vi "Motor Overheat detection.vi"() -> (0 "Array":string[](array[string]), 1 "Cascade Sensor":bool, 2 "Rhino Sensors":bool, 3 "Drivebase Sensors":bool)   [LabVIEW 2018]
uses:
  <vilib>/ptbypt/NI_PtbyPt.lvlib
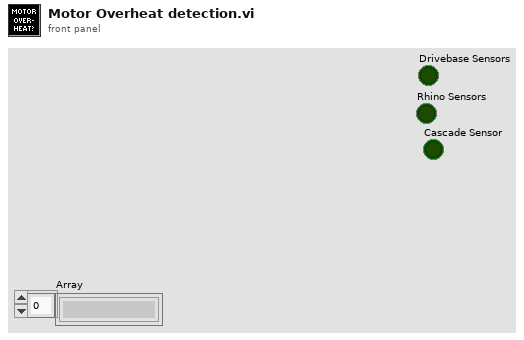
[diagram p1: front panel]
types:
  T1 = typedef "WPI_MotorControlDeviceRef.ctl" = cluster{"DeviceStatus":errorcluster, "Type":T2, "PWM":cluster{"PWM Channel":T3, "DeadBand":T4}, "CAN":cluster{"Device Number":u8, "SetOutput VI Ref":variant, "GetOutput VI Ref":variant, "Enable VI Ref":variant, "Disable VI Ref":variant, "Data":variant}, "Invert":bool, "DIO PWM":cluster{"PWM \"Enable\" Channel":T3, "DIOChannel":T5, "PWM Rate":dbl}}
  T2 = typedef "WPI_MotorControlType.ctl" = enum16{"PWM", "CAN", "DIO PWM"}
  T3 = typedef "FPGA_DIOPWMChannel.ctl" = enum8{"PWM 0", "PWM 1", "PWM 2", "PWM 3", "PWM 4", "PWM 5", "PWM 6", "PWM 7", "PWM 8", "PWM 9", "PWM MXP 0", "PWM MXP 1", "PWM MXP 2", "PWM MXP 3", "PWM MXP 4", "PWM MXP 5", "PWM MXP 6", "PWM MXP 7", "PWM MXP 8", "PWM MXP 9", "Invalid"}
  T4 = typedef "WPI_PWMDeadband.ctl" = cluster{"Name":string, "maxPositivePwm":i32, "minPositivePwm":i32, "centerPwm":i32, "maxNegativePwm":i32, "minNegativePwm":i32, "angularRange":u16}
  T5 = typedef "FPGA_DIOChannel.ctl" = enum8{"DIO 0", "DIO 1", "DIO 2", "DIO 3", "DIO 4", "DIO 5", "DIO 6", "DIO 7", "DIO 8", "DIO 9", "DIO MXP 0", "DIO MXP 1", "DIO MXP 2", "DIO MXP 3", "DIO MXP 4", "DIO MXP 5", "DIO MXP 6", "DIO MXP 7", "DIO MXP 8", "DIO MXP 9", "DIO MXP 10", "DIO MXP 11", "DIO MXP 12", "DIO MXP 13", "DIO MXP 14", "DIO MXP 15", "SPI Port CS1", "SPI Port CS2", "SPI Port CS3", "SPI Port MISO", "SPI Port MOSI", "Invalid"}
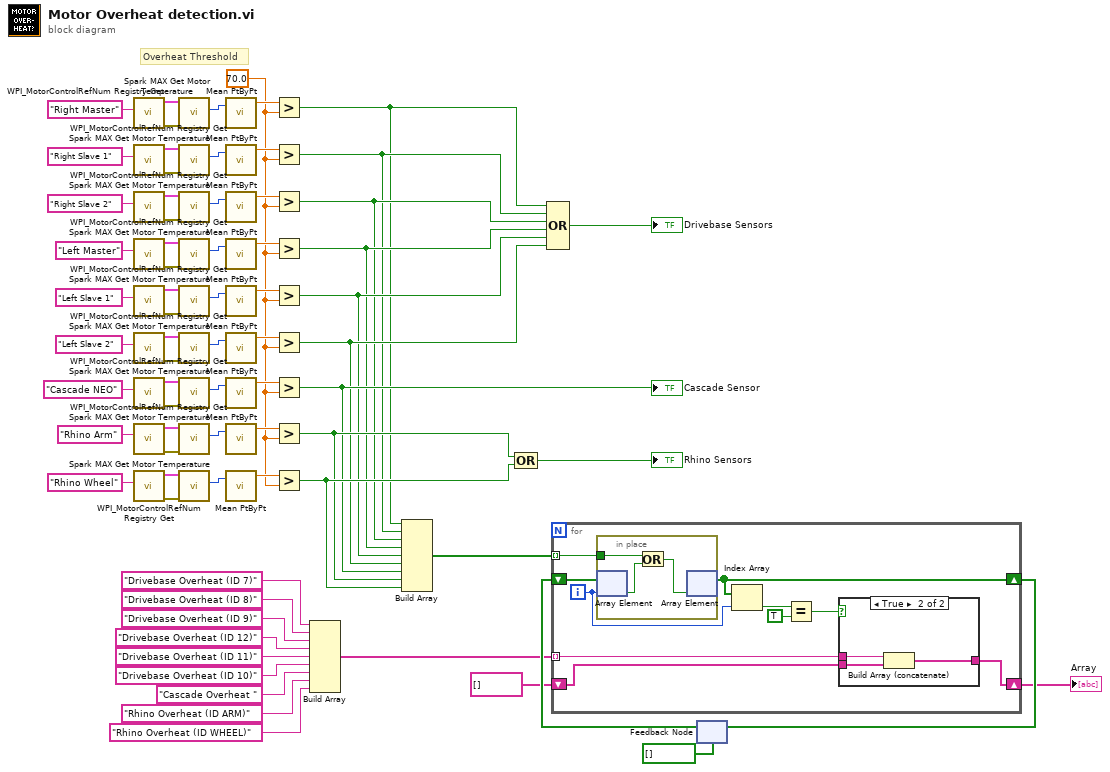
[diagram p0: block diagram]
diagram:
  w28 = 70.0 ("y")
  # "Overheat Threshold"
  n1 = call <vilib>:"WPI_MotorControlRefNum Registry Get.vi"("refnum name"="Right Master") -> ("error out"=w61:errorcluster, "MotorControlDevRef"=w64:T1)  [unwired: 9 in]
  n2 = call <vilib>:"WPI_MotorControlRefNum Registry Get.vi"("refnum name"="Right Slave 1") -> ("error out"=w59:errorcluster, "MotorControlDevRef"=w60:T1)  [unwired: 9 in]
  n3 = call <vilib>:"WPI_MotorControlRefNum Registry Get.vi"("refnum name"="Right Slave 2") -> ("error out"=w57:errorcluster, "MotorControlDevRef"=w58:T1)  [unwired: 9 in]
  n4 = call <vilib>:"WPI_MotorControlRefNum Registry Get.vi"("refnum name"="Left Master") -> ("error out"=w55:errorcluster, "MotorControlDevRef"=w56:T1)  [unwired: 9 in]
  n5 = call <vilib>:"WPI_MotorControlRefNum Registry Get.vi"("refnum name"="Left Slave 1") -> ("error out"=w53:errorcluster, "MotorControlDevRef"=w54:T1)  [unwired: 9 in]
  n6 = call <vilib>:"WPI_MotorControlRefNum Registry Get.vi"("refnum name"="Left Slave 2") -> ("error out"=w51:errorcluster, "MotorControlDevRef"=w52:T1)  [unwired: 9 in]
  n7 = call <vilib>:"WPI_MotorControlRefNum Registry Get.vi"("refnum name"="Cascade NEO") -> ("error out"=w49:errorcluster, "MotorControlDevRef"=w50:T1)  [unwired: 9 in]
  n8 = call <vilib>:"WPI_MotorControlRefNum Registry Get.vi"("refnum name"="Rhino Arm") -> ("error out"=w47:errorcluster, "MotorControlDevRef"=w48:T1)  [unwired: 9 in]
  n9 = call <vilib>:"WPI_MotorControlRefNum Registry Get.vi"("refnum name"="Rhino Wheel") -> ("error out"=w63:errorcluster, "MotorControlDevRef"=w62:T1)  [unwired: 9 in]
  n10 = call <vilib>:"Spark MAX Get Motor Temperature.vi"("error in (no error)"=w61, "MotorControlDevRef in"=w64) -> ("Motor Temperature"=w46:u8)  [unwired: 6 in, 3 out]
  n11 = call <vilib>:"Spark MAX Get Motor Temperature.vi"("error in (no error)"=w59, "MotorControlDevRef in"=w60) -> ("Motor Temperature"=w38:u8)  [unwired: 6 in, 3 out]
  n12 = call <vilib>:"Spark MAX Get Motor Temperature.vi"("error in (no error)"=w57, "MotorControlDevRef in"=w58) -> ("Motor Temperature"=w39:u8)  [unwired: 6 in, 3 out]
  n13 = call <vilib>:"Spark MAX Get Motor Temperature.vi"("error in (no error)"=w55, "MotorControlDevRef in"=w56) -> ("Motor Temperature"=w40:u8)  [unwired: 6 in, 3 out]
  n14 = call <vilib>:"Spark MAX Get Motor Temperature.vi"("error in (no error)"=w53, "MotorControlDevRef in"=w54) -> ("Motor Temperature"=w41:u8)  [unwired: 6 in, 3 out]
  n15 = call <vilib>:"Spark MAX Get Motor Temperature.vi"("error in (no error)"=w51, "MotorControlDevRef in"=w52) -> ("Motor Temperature"=w42:u8)  [unwired: 6 in, 3 out]
  n16 = call <vilib>:"Spark MAX Get Motor Temperature.vi"("error in (no error)"=w49, "MotorControlDevRef in"=w50) -> ("Motor Temperature"=w43:u8)  [unwired: 6 in, 3 out]
  n17 = call <vilib>:"Spark MAX Get Motor Temperature.vi"("error in (no error)"=w47, "MotorControlDevRef in"=w48) -> ("Motor Temperature"=w44:u8)  [unwired: 6 in, 3 out]
  n18 = call <vilib>:"Spark MAX Get Motor Temperature.vi"("error in (no error)"=w63, "MotorControlDevRef in"=w62) -> ("Motor Temperature"=w45:u8)  [unwired: 6 in, 3 out]
  n19 = call <vilib>:"Mean PtByPt.vi"("x"=w46) -> ("mean"=w37:dbl)  [unwired: 3 in, 1 out]
  n20 = call <vilib>:"Mean PtByPt.vi"("x"=w38) -> ("mean"=w36:dbl)  [unwired: 3 in, 1 out]
  n21 = call <vilib>:"Mean PtByPt.vi"("x"=w39) -> ("mean"=w35:dbl)  [unwired: 3 in, 1 out]
  n22 = call <vilib>:"Mean PtByPt.vi"("x"=w40) -> ("mean"=w34:dbl)  [unwired: 3 in, 1 out]
  n23 = call <vilib>:"Mean PtByPt.vi"("x"=w41) -> ("mean"=w33:dbl)  [unwired: 3 in, 1 out]
  n24 = call <vilib>:"Mean PtByPt.vi"("x"=w42) -> ("mean"=w32:dbl)  [unwired: 3 in, 1 out]
  n25 = call <vilib>:"Mean PtByPt.vi"("x"=w43) -> ("mean"=w31:dbl)  [unwired: 3 in, 1 out]
  n26 = call <vilib>:"Mean PtByPt.vi"("x"=w44) -> ("mean"=w30:dbl)  [unwired: 3 in, 1 out]
  n27 = call <vilib>:"Mean PtByPt.vi"("x"=w45) -> ("mean"=w29:dbl)  [unwired: 3 in, 1 out]
  n28 = Greater?(x=w37, y=w28) -> (0:w1:bool)
  n29 = Greater?(x=w36, y=w28) -> (0:w2:bool)
  n30 = Greater?(x=w35, y=w28) -> (0:w3:bool)
  n31 = Greater?(x=w34, y=w28) -> (0:w4:bool)
  n32 = Greater?(x=w33, y=w28) -> (0:w5:bool)
  n33 = Greater?(x=w32, y=w28) -> (0:w6:bool)
  n34 = Greater?(x=w31, y=w28) -> (0:w7:bool)
  "Cascade Sensor" <- w7
  n35 = Greater?(x=w30, y=w28) -> (0:w8:bool)
  n36 = Greater?(x=w29, y=w28) -> (0:w9:bool)
  n37 = Build Array("Drivebase Overheat (ID 7)" ("refnum name"), "Drivebase Overheat (ID 8)" ("refnum name"), "Drivebase Overheat (ID 9)" ("refnum name"), "Drivebase Overheat (ID 12)" ("refnum name"), "Drivebase Overheat (ID 11)" ("refnum name"), "Drivebase Overheat (ID 10)" ("refnum name"), "Cascade Overheat " ("refnum name"), "Rhino Overheat (ID ARM)" ("refnum name"), "Rhino Overheat (ID WHEEL)" ("refnum name")) -> (w12:string[])
  n38 = Build Array(w1, w2, w3, w4, w5, w6, w7, w8, w9) -> (w24:bool[])
  n39 = Compound Arithmetic op=OR(w8, w9) -> (→"Rhino Sensors":bool)
  n40 = Compound Arithmetic op=OR(w1, w2, w3, w4, w5, w6) -> (→"Drivebase Sensors":bool)
  n41 = feedback #1(bool[] [] ("appended array")) -> (w23:bool[])
  n42 = for {
    tunnel: w24 -> [w82] mode=indexing
    shift-right: [w81] -> w25
    shift-left: w23 -> [w83]
    tunnel: w12 -> [w75] mode=indexing
    shift-right: [w74] -> w10
    shift-left: string[] [] -> [w76]
    i -> [w80]
    n43 = in-place {
      in-place-border: w82 -> [w86]
      n44 = in-place-array #2(w83, w80) -> (w84:bool)
      n45 = Or(x=w86, y=w84) -> (x .or. y?=w85:bool)
      n46 = in-place-array #2(w85) -> (w81:bool[])  [unwired: 1 out]
    }
    n47 = Index Array(array=w81, index=w80) -> (element=w79:bool)
    n48 = Equal?(x=w79, y=TRUE) -> (x = y?=w77:bool)
    n49 = case shown="True" w77 {
      tunnel: w76 -> [w87 w90]
      tunnel: w75 -> [_ w89]
      tunnel: [w87 w88] -> w74
      frame False {
      }
      frame True {
        n50 = Build Array (concatenate)(w89, w90) -> (w88:string[])
      }
    }
  }
  "Array" <- w10
  n51 = feedback-in #1(w25) -> ()
